vi "测试.vi"() -> ()   [LabVIEW 2018]
panel:
  out "布尔":bool
  in  "停止":bool
  in  "P":dbl=1.0
  out "Output Value":dbl format="%.2f"
  in  "IP Port":string="22222"
  in  "IP Address":string="192.168.0.3"
  in  "Host COM Port":u16(ring) items=["COM1", "COM2"]
  in  "Host Target communication":u16(ring) items=["TCP/IP", "RS232"]
  in  "Application filename":string="simpleCylinder1"
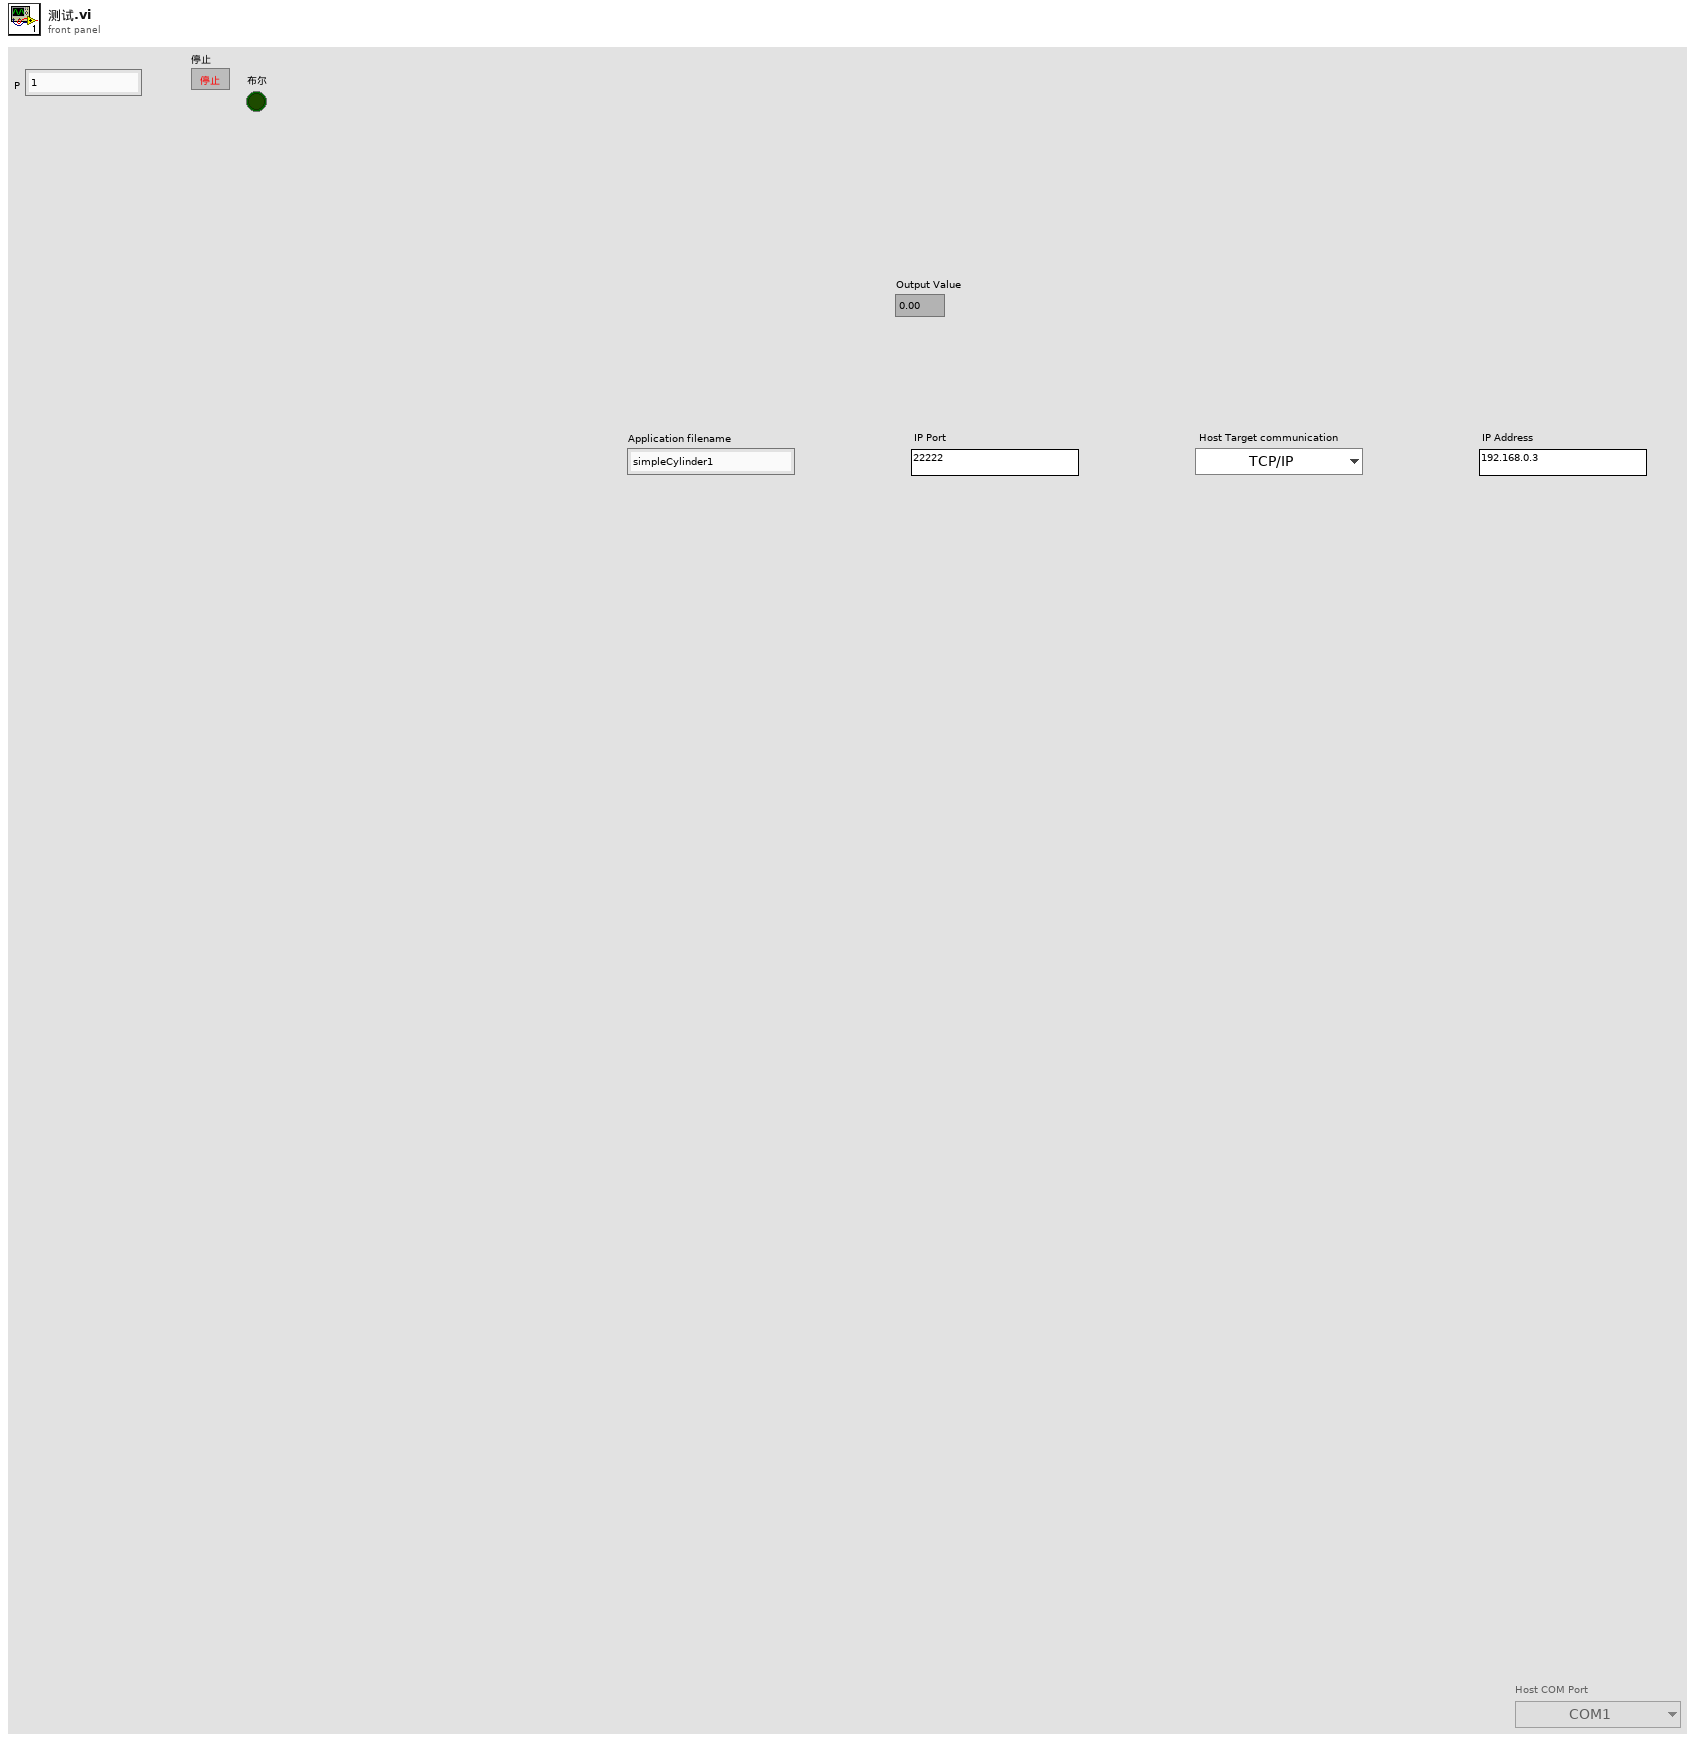
[diagram p1: front panel]
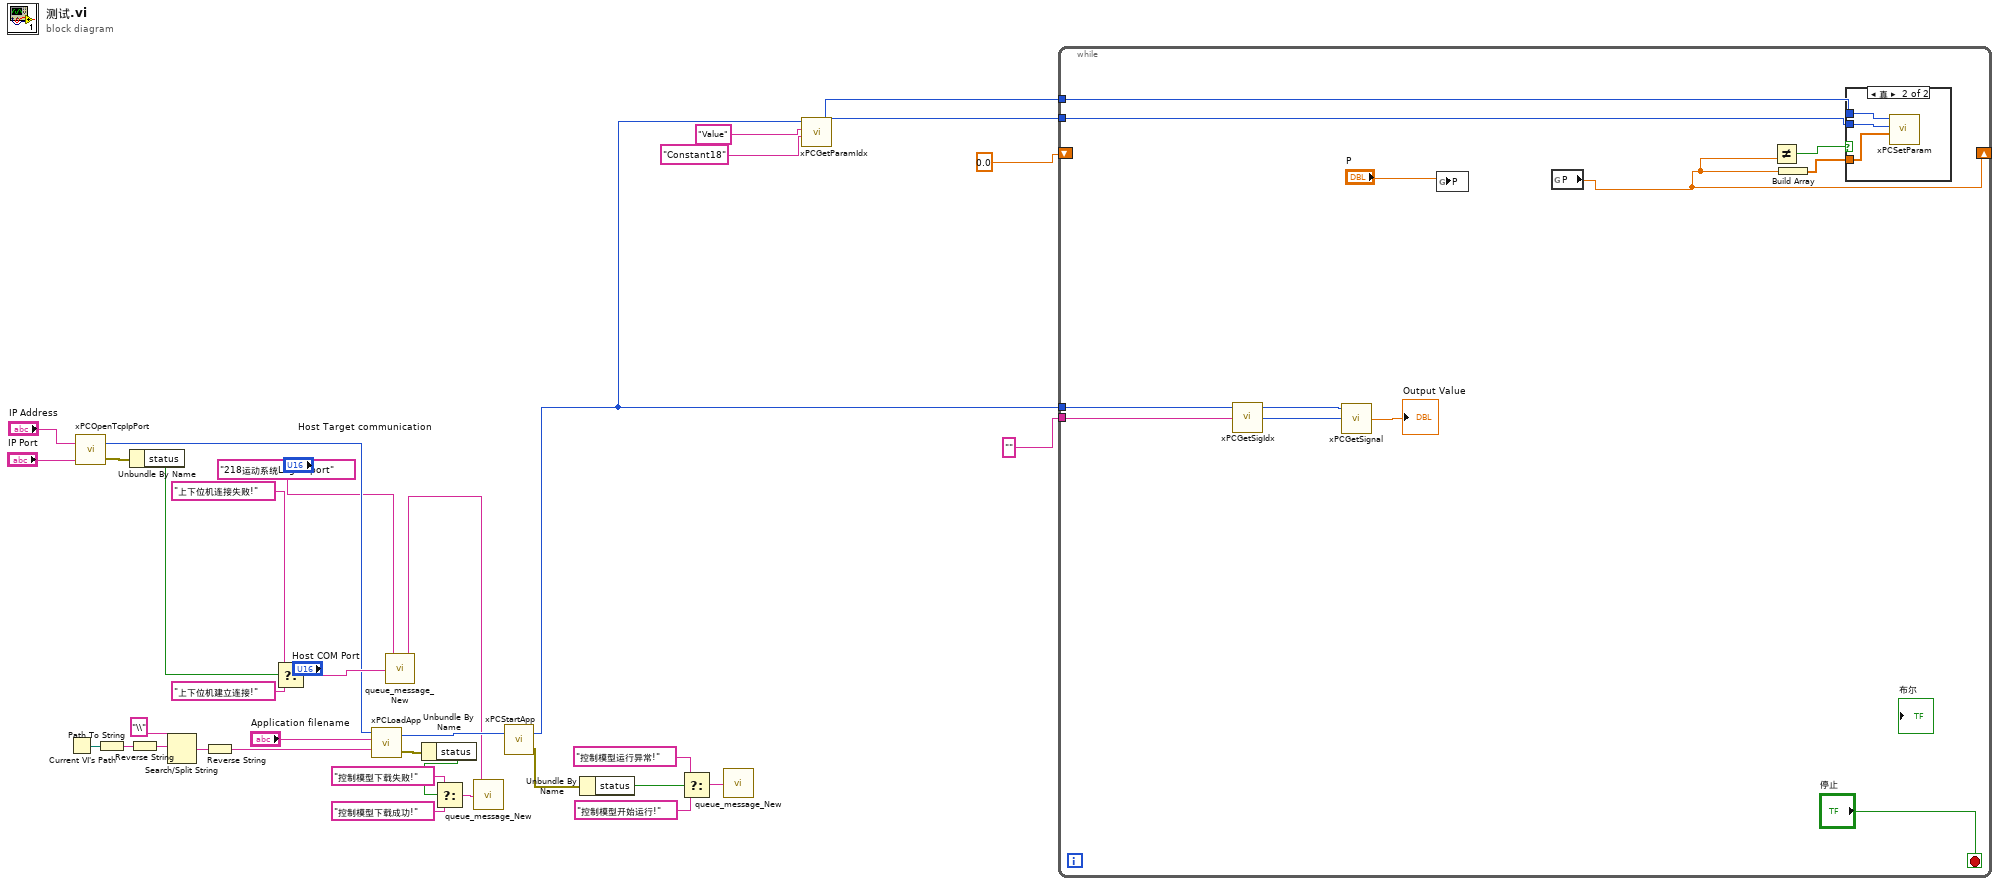
[diagram p0: block diagram]
diagram:
  n1 = Current VI's Path() -> (path=w29:path)
  n2 = call "xPCOpenTcpIpPort.vi"("port"="IP Port", "address"="IP Address") -> ("error out"=w16:errorcluster, "Port"=w17:i32)
  n3 = Path To String(path=w29) -> (string=w31:string)
  n4 = Unbundle By Name(w16) -> ("status"=w27:bool)
  n5 = Reverse String(1:w31) -> (0:w33:string)
  n6 = Search/Split String(string=w33, search string/char (-)="\\" ("search char (-)")) -> (match + rest of string=w32:string)  [unwired: 1 in, 2 out]
  n7 = Reverse String(1:w32) -> (0:w34:string)
  n8 = Select(t="上下位机连接失败!" ("message"), s=w27, f="上下位机建立连接!" ("message")) -> (s? t:f=w24:string)
  n9 = call "xPCLoadApp.vi"("pathstr"=w34, "filename"="Application filename", "port"=w17) -> ("error out"=w18:errorcluster, "port copy"=w28:i32)  [unwired: 1 in]
  n10 = call "queue_message_New.vi"("message"=w24, "queue_name"="218运动系统Log Report") -> ("queue_name_copy"=w23:string)  [unwired: 1 in, 1 out]
  n11 = Unbundle By Name(w18) -> ("status"=w21:bool)
  n12 = Select(t="控制模型下载失败!" ("message"), s=w21, f="控制模型下载成功!" ("message")) -> (s? t:f=w22:string)
  n13 = call "queue_message_New.vi"("message"=w22, "queue_name"=w23) -> ()  [unwired: 1 in, 2 out]
  n14 = call "xPCStartApp.vi"("port"=w28) -> ("error out"=w8:errorcluster, "port copy"=w2:i32)  [unwired: 1 in]
  n15 = Unbundle By Name(w8) -> ("status"=w11:bool)
  n16 = Select(t="控制模型运行异常!" ("message"), s=w11, f="控制模型开始运行!" ("message")) -> (s? t:f=w10:string)
  n17 = call "queue_message_New.vi"("message"=w10) -> ()  [unwired: 2 in, 2 out]
  n18 = call "xPCGetParamIdx.vi"("blockpath"="Constant18" ("pathstr"), "parametername"="Value" ("filename"), "port"=w2) -> ("identifier"=w4:i32, "port copy"=w5:i32)  [unwired: 1 in, 1 out]
  n19 = while {
    tunnel: w5 -> [w44]
    tunnel: w4 -> [w43]
    shift-right: [w42] -> _
    shift-left: 0.0 -> [_]
    tunnel: "" ("blockpath") -> [w38]
    tunnel: w2 -> [w37]
    stop <- "停止" stop-if-true
    n20 = call "xPCGetSigIdx.vi"("blockpath"=w38, "port"=w37) -> ("identifier"=w40:i32, "port copy"=w39:i32)  [unwired: 1 in, 1 out]
    n21 = call "xPCGetSignal.vi"("signal"=w40, "port"=w39) -> ("Output Value"=→"Output Value":dbl)  [unwired: 1 in, 2 out]
    n22 = global write "全局 1.vi" "P"("P") -> ()
    n23 = global read "全局 1.vi" "P"() -> (w42:dbl)
    n24 = Not Equal?(y=w42) -> (x != y?=w46:bool)  [unwired: 1 in]
    n25 = Build Array(w42) -> (w47:dbl[])
    n26 = case shown="真" w46 {
      tunnel: w44 -> [_ w50]
      tunnel: w43 -> [_ w49]
      tunnel: w47 -> [_ w48]
      frame False {
      }
      frame True {
        n27 = call "xPCSetParam.vi"("value"=w48, "index"=w49, "port"=w50) -> ()  [unwired: 1 in, 2 out]
      }
    }
  }
